vi "StartUIProgress.vi"(8 "error in (no error)":errorcluster, 11 "Progress in":refnum<class "Progress.lvclass">) -> (0 "error out":errorcluster, 3 "Progress out":refnum<class "Progress.lvclass">)   [LabVIEW 2021, in "Progress.lvlib" / "Progress.lvclass"]
uses:
  Progress.lvclass
  UI_Progress.vi
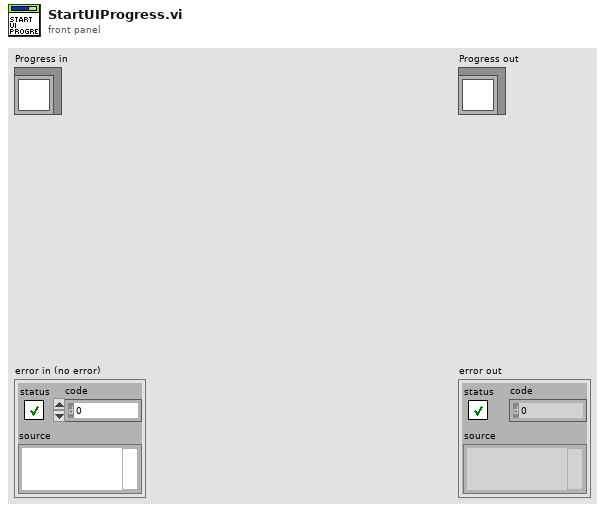
[diagram p1: front panel]
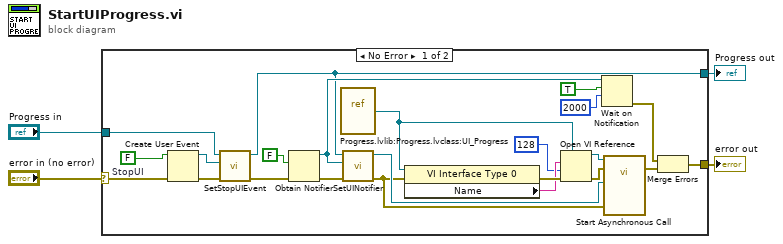
[diagram p0: block diagram]
diagram:
  n1 = case shown="No Error" "error in (no error)" {
    selector: "error in (no error)" -> [w17 w29]
    tunnel: [w22 w29] -> w3
    tunnel: [w12 w28] -> w1
    tunnel: "Progress in" -> [w11 w28]
    frame No Error {
      w16 = FALSE  # StopUI
      n2 = Create User Event(user event datatype=w16, error in=w17) -> (user event=w13:refnum<user-event>, error out=w15:errorcluster)
      n3 = call "SetStopUIEvent.vi"("error in (no error)"=w15, "StopUIEvent"=w13, "Progress in"=w11) -> ("error out"=w14:errorcluster, "Progress out"=w12:refnum<class "Progress.lvclass">)  [unwired: 7 in]
      n4 = Obtain Notifier(notification data type=FALSE, error in (no error)=w14) -> (notifier out=w23:refnum<notifier>, error out=w24:errorcluster)  [unwired: 2 in, 1 out]
      n5 = vi-ref "Progress.lvlib:Progress.lvclass:UI_Progress.vi"() -> (w7:refnum<vi>)
      n6 = call "SetUINotifier.vi"("error in (no error)"=w24, "UINotifier"=w23, "Progress in"=w12) -> ("error out"=w18:errorcluster, "Progress out"=w25:refnum<class "Progress.lvclass">)  [unwired: 7 in]
      n7 = property class="VI Interface Type 0"(reference=w7, error in=w18) -> (error out=w8:errorcluster, "Name"=w6:string)  [unwired: 1 out]
      n8 = Open VI Reference(type specifier VI Refnum (for type only)=w7, vi path=w6, options=128, error in (no error)=w8) -> (vi reference=w9:refnum<vi>, error out=w10:errorcluster)  [unwired: 2 in]
      n9 = Wait on Notification(notifier=w23, ignore previous (F)=TRUE, timeout in ms (-1)=2000) -> (error out=w21:errorcluster)  [unwired: 1 in, 3 out]
      n10 = call-by-ref "Start Asynchronous Call"(reference=w9, error in=w10, 8:"error in (no error)"=w18, "Progress in"=w25) -> (error out=w27:errorcluster)  [unwired: 8 in, 3 out]
      n11 = Merge Errors(w21, w27) -> (w22:errorcluster)
    }
    frame Error {
    }
  }
  "error out" <- w3
  "Progress out" <- w1
